vi "Delete Parameters .vi"(0 "VISA IN":refnum<visa-resource-name>, 1 "Delete All?":bool, 2 "Measurement Name":string, 5 "error in":errorcluster, 7 "Channel":i32=1) -> (14 "VISA Out":refnum<visa-resource-name>, 19 "error out":errorcluster)   [LabVIEW 2018, in "PNA-X.lvlib"]
uses:
  PNA-X.lvlib
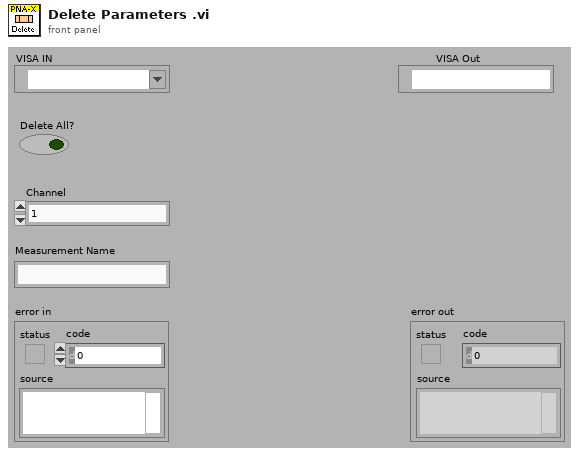
[diagram p1: front panel]
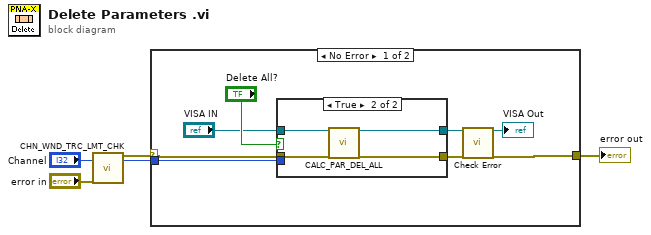
[diagram p0: block diagram]
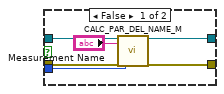
[diagram p2: hidden frame]
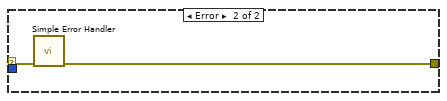
[diagram p3: hidden frame]
diagram:
  n1 = call "CHN_WND_TRC_LMT_CHK.vi"("Channel"="Channel", "error in"="error in") -> ("error out"=w2:errorcluster, "Channel"=w1:i32)  [unwired: 13 in, 3 out]
  n2 = case shown="No Error" w2 {
    selector: w2 -> [w8 w25]
    tunnel: [w13 w24] -> w4
    tunnel: w1 -> [w6 _]
    frame No Error {
      n3 = case shown="True" "Delete All?" {
        tunnel: "VISA IN" -> [w16 w23]
        tunnel: [w19 w22] -> w9
        tunnel: w8 -> [w17 w21]
        tunnel: [w18 w20] -> w7
        tunnel: w6 -> [w15 _]
        frame False {
          n4 = call "CALC_PAR_DEL_NAME_M.vi"("VISA IN"=w16, "Measurement Name"="Measurement Name", "error in"=w17, "Channel"=w15) -> ("VISA Out"=w19:refnum<visa-resource-name>, "error out"=w18:errorcluster)  [unwired: 14 in]
        }
        frame True {
          n5 = call "CALC_PAR_DEL_ALL.vi"("VISA IN"=w23, "error in"=w21) -> ("VISA Out"=w22:refnum<visa-resource-name>, "error out"=w20:errorcluster)  [unwired: 16 in]
        }
      }
      n6 = call "Check Error.vi"("VISA Resource Name"=w9, "error in (no error)"=w7) -> ("dup VISA session"=→"VISA Out":refnum<visa-resource-name>, "error out"=w13:errorcluster)  [unwired: 16 in]
    }
    frame Error {
      n7 = call <vilib>:"Simple Error Handler.vi"("error in (no error)"=w25) -> ("error out"=w24:errorcluster)  [unwired: 4 in, 4 out]
    }
  }
  "error out" <- w4
